vi "MS Operation IOP Ctrl.vi"(6 "PID Cluster":T3={"L1 to L4 PID Cluster"={"L1 PID Gains"={"Kp"=0.005, "Kd"=0.5, "Ki"=0.0005}, "L2 PID Gains"={"Kp"=0.01, "Kd"=1.0, "Ki"=0.005}, "L3 PID Gains"={"Kp"=0.05, "Kd"=1.0, "Ki"=0.0005}, "L4 PID Gains"={"Kp"=0.1, "Kd"=0.1, "Ki"=0.0005}}, "Stage PID Cluster"={"Stage Z PID"={"Kp"=0.0005, "Kd"=0.001, "Ki"=0.0}, "Stage Y PID"={"Kp"=0.0003, "Kd"=0.01, "Ki"=0.0}, "Stage X PID"={"Kp"=0.0003, "Kd"=0.01, "Ki"=0.0}}, "OCT Z PID Gains"={"Kp"=0.0003, "Kd"=0.0001, "Ki"=0.01}}, 8 "error in":errorcluster, 9 "Offset Home 2 RCM":dbl[](array[numeric])=[0.0, 0.0, 0.0, 0.0], 10 "Prev Posit Cluster":T2={"Prev L1 to L4 Posit"=[-0.5319, -0.035669172703475985, -2.0566170657346783, 0.9099264705882353], "Prev Stage Posit"=[6.002553885707208, 5.996566124542428, 5.995469940427586], "Prev OCT Z Posit"=-0.0}, 11 "FPGA VI Reference In":refnum<k20>) -> (0 "error out":errorcluster, 2 "Last Posit Cluster":T1={"Last L1 to L4 Posit"=[0.0, 0.0, 0.0, 0.0], "Last Stage Posit"=[6.0, 6.0, 6.0], "Last OCT Z Posit"=0.0}, 3 "FPGA VI Reference Out":refnum<k20>)   [LabVIEW 2016]
uses:
  <vilib>/Platform/TimedLoop/XDataNode/timing_clust.ctl
  <vilib>/Platform/TimedLoop/XDataNode/nitl_modes.ctl
  <vilib>/Platform/TimedLoop/XDataNode/wakeup.ctl
  Global Variables.vi
  <vilib>/platform/TimedLoop/XDataNode/XDataNode.xnode
  <vilib>/Platform/TimedLoop/XDataNode/XDNodeRunTimeDep.lvlib
  Library/KevinLibraryAll/labview/KevLib01.lvlib
panel:
  out "L1 to L4 Remote cmd":sgl[](array[numeric])
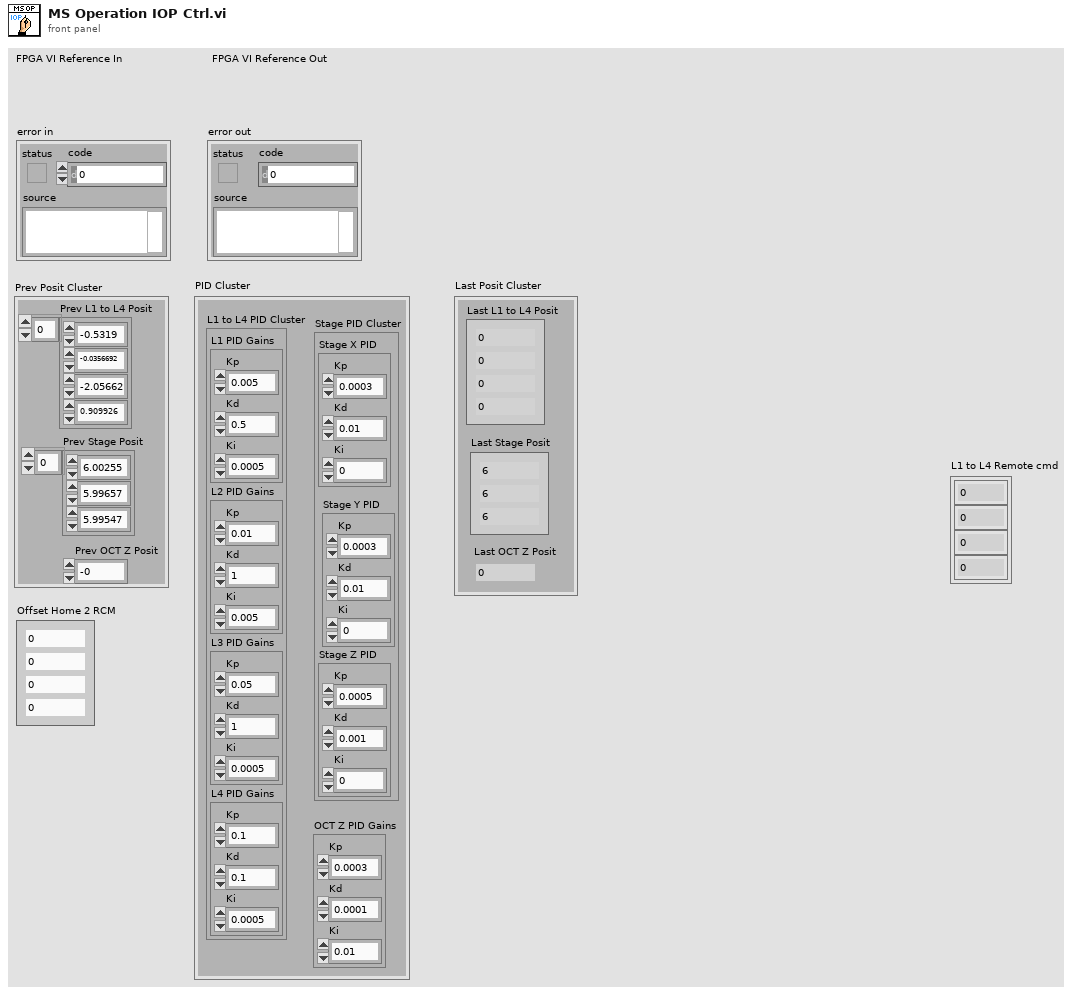
[diagram p1: front panel]
types:
  T1 = cluster{"Last L1 to L4 Posit":dbl[], "Last Stage Posit":dbl[], "Last OCT Z Posit":dbl}
  T2 = cluster{"Prev L1 to L4 Posit":dbl[], "Prev Stage Posit":dbl[], "Prev OCT Z Posit":dbl}
  T3 = cluster{"L1 to L4 PID Cluster":cluster{"L1 PID Gains":cluster{"Kp":dbl, "Kd":dbl, "Ki":dbl}, "L2 PID Gains":cluster{"Kp":dbl, "Kd":dbl, "Ki":dbl}, "L3 PID Gains":cluster{"Kp":dbl, "Kd":dbl, "Ki":dbl}, "L4 PID Gains":cluster{"Kp":dbl, "Kd":dbl, "Ki":dbl}}, "Stage PID Cluster":cluster{"Stage Z PID":cluster{"Kp":dbl, "Kd":dbl, "Ki":dbl}, "Stage Y PID":cluster{"Kp":dbl, "Kd":dbl, "Ki":dbl}, "Stage X PID":cluster{"Kp":dbl, "Kd":dbl, "Ki":dbl}}, "OCT Z PID Gains":cluster{"Kp":dbl, "Kd":dbl, "Ki":dbl}}
  T4 = typedef "XDNodeRunTimeDep.lvlib/timing_clust.ctl" = cluster{"Expected End [f-1]":u64, "Actual End [f-1]":u64, "Finished Late? [f-1]":bool, "Expected End [i-1]":u64, "Actual End [i-1]":u64, "Finished Late? [i-1]":bool, "Expected Start [i]":u64, "Actual Start [i]":u64, "Expected Start [f]":u64, "Actual Start [f]":u64, "Source Name":string, "Structure Name":string, "Period":i64, "Deadline":i64, "Offset":i64, "Start":i64, "Priority":i32, "Timeout":i32, "Mode":T5, "Wakeup Reason":T6, "Error":errorcluster, "Source Type":string, "Secondary Source Type":string, "Global End Time":u64, "Global Start Time":u64, "Frame Duration":u64, "Iteration Duration":u64, "Assigned CPU":i32, "I/O Scan Engine Mode":u32}
  T5 = typedef "XDNodeRunTimeDep.lvlib/nitl_modes.ctl" = enum32{"No Change", "Process missed periods, maintain original phase", "Discard missed periods, maintain original phase", "Process missed periods, ignore original phase", "Discard missed periods, ignore original phase"}
  T6 = typedef "XDNodeRunTimeDep.lvlib/wakeup.ctl" = enum32{"Normal", "Aborted", "Asynchronous wakeup", "Timing source error", "Timed loop error", "Timeout"}
  T7 = cluster{"L1 PID Gains":cluster{"Kp":dbl, "Kd":dbl, "Ki":dbl}, "L2 PID Gains":cluster{"Kp":dbl, "Kd":dbl, "Ki":dbl}, "L3 PID Gains":cluster{"Kp":dbl, "Kd":dbl, "Ki":dbl}, "L4 PID Gains":cluster{"Kp":dbl, "Kd":dbl, "Ki":dbl}}
  T8 = cluster{"Stage Z PID":cluster{"Kp":dbl, "Kd":dbl, "Ki":dbl}, "Stage Y PID":cluster{"Kp":dbl, "Kd":dbl, "Ki":dbl}, "Stage X PID":cluster{"Kp":dbl, "Kd":dbl, "Ki":dbl}}
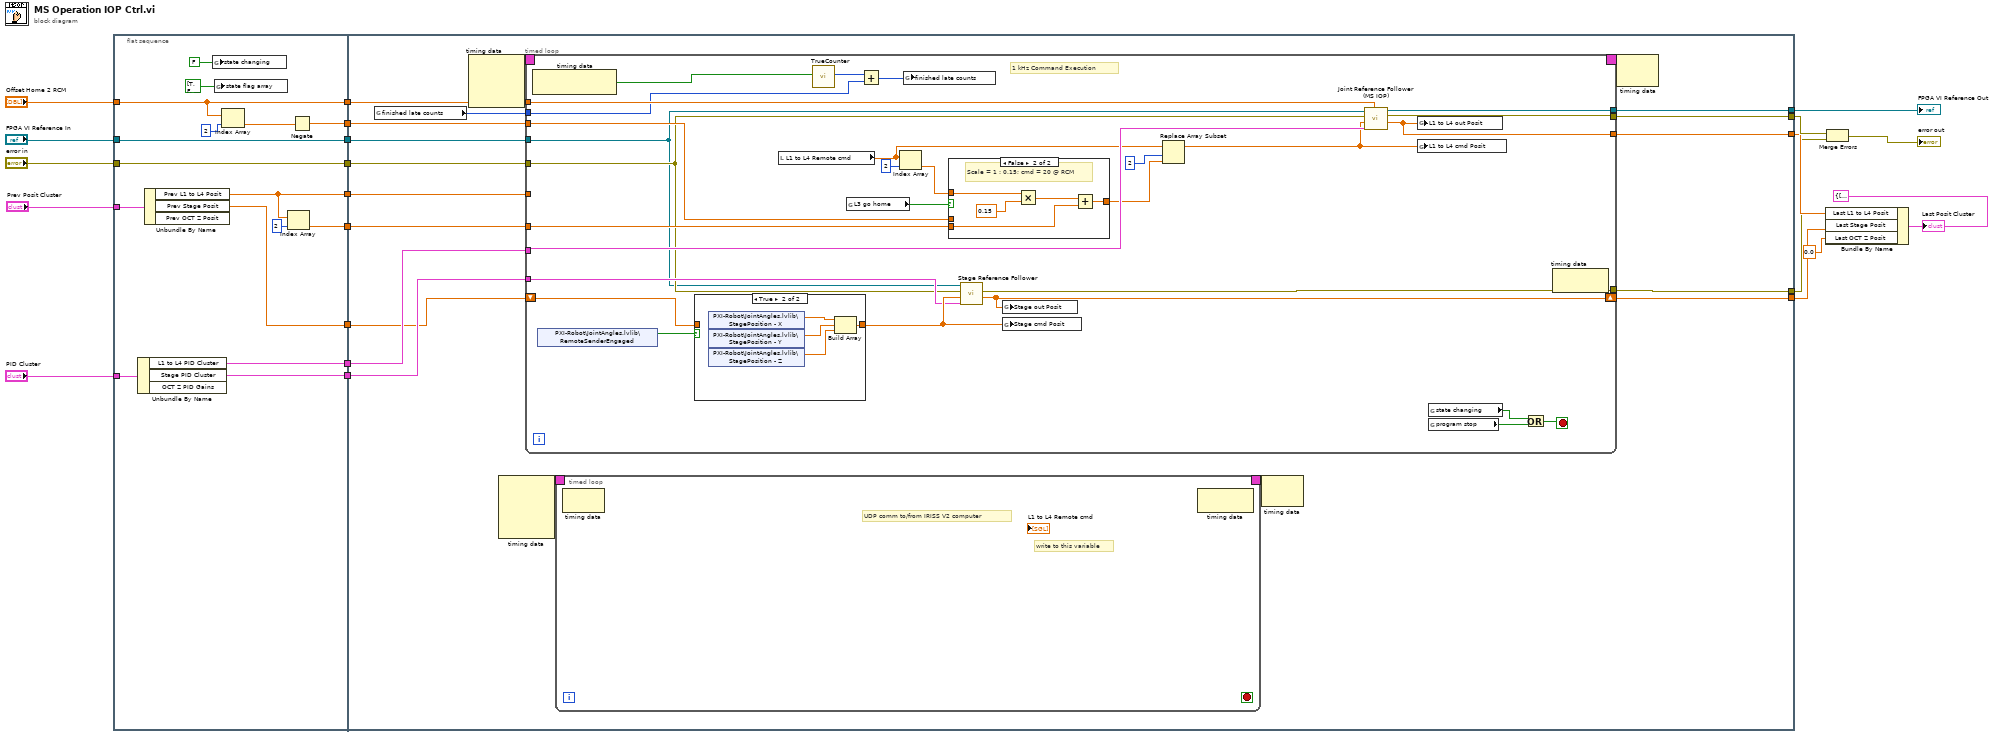
[diagram p0: block diagram]
diagram:
  n1 = flat-sequence {
    tunnel: [w37] -> w23
    tunnel: "FPGA VI Reference In" -> [w37]
    tunnel: [w36] -> w21
    tunnel: "error in" -> [w36]
    tunnel: [w29] -> w19
    tunnel: "Offset Home 2 RCM" -> [w29]
    tunnel: "Prev Posit Cluster" -> [w25]
    tunnel: [w34] -> w16
    tunnel: "PID Cluster" -> [w33]
    tunnel: [w32] -> w14
    tunnel: [w31] -> w13
    tunnel: [w27] -> w12
    tunnel: [w26] -> w3
    tunnel: [w24] -> w2
    tunnel: w23 -> [w43]
    tunnel: w21 -> [w42]
    tunnel: w19 -> [w56]
    tunnel: w16 -> [w55]
    tunnel: w14 -> [w54]
    tunnel: w13 -> [w53]
    tunnel: w12 -> [w52]
    tunnel: [w51] -> w8
    tunnel: [w50] -> w9
    tunnel: [w44] -> w6
    tunnel: [w45] -> w5
    tunnel: [w49] -> w4
    tunnel: w3 -> [w48]
    tunnel: w2 -> [w46]
    frame #0 {
      n2 = Unbundle By Name(w33) -> ("L1 to L4 PID Cluster"=w32:T7, "Stage PID Cluster"=w26:T8)  [unwired: 1 out]
      n3 = Unbundle By Name(w25) -> ("Prev L1 to L4 Posit"=w34:dbl[], "Prev Stage Posit"=w24:dbl[])  [unwired: 1 out]
      n4 = global write "Global Variables.vi" "state changing"(FALSE ("state changing")) -> ()
      n5 = global write "Global Variables.vi" "state flag array"(bool[] [TRUE, FALSE, FALSE, FALSE, FALSE, FALSE, FALSE, FALSE, FALSE] ("state flag array")) -> ()
      n6 = Index Array(array=w29, index=2) -> (element=w28:dbl)
      n7 = Index Array(array=w34, index=2) -> (element=w31:dbl)
      n8 = Negate(x=w28) -> (-x=w27:dbl)
    }
    frame #1 {
      n9 = global read "Global Variables.vi" "finished late counts"() -> (w47:u16)
      n10 = node-c288() -> (w58:T4)  [unwired: 3 in]
      n11 = node-c288() -> (w41:T4)  [unwired: 4 in]
      n12 = timed-loop {
        timing: w58 -> [_]
        timing-out: [_] -> w57
        tunnel: w43 -> [w69]
        tunnel: w42 -> [w70]
        tunnel: w56 -> [w86]
        tunnel: w55 -> [_]
        tunnel: w54 -> [w84]
        tunnel: w53 -> [w83]
        tunnel: w52 -> [w80]
        tunnel: [w79] -> w51
        tunnel: [w78] -> w50
        tunnel: [w77] -> w49
        tunnel: w48 -> [w75]
        tunnel: w47 -> [w71]
        shift-right: [w67] -> w45
        shift-left: w46 -> [w68]
        tunnel: [w64] -> w44
        stop <- w91 stop-if-true
        # "1 kHz Command Execution"
        n13 = node-c288() -> (w74:bool)  [unwired: 1 in]
        n14 = shared-variable "PXI-Robot\\JointAngles.lvlib\\RemoteSenderEngaged"() -> (w66:bool)  [unwired: 1 in, 1 out]
        n15 = case shown="True" w66 {
          tunnel: [w92 w96] -> w85
          tunnel: w68 -> [w92 _]
          frame False {
          }
          frame True {
            n16 = shared-variable "PXI-Robot\\JointAngles.lvlib\\StagePosition - X"() -> (w93:dbl)  [unwired: 1 in, 1 out]
            n17 = shared-variable "PXI-Robot\\JointAngles.lvlib\\StagePosition - Y"() -> (w94:dbl)  [unwired: 1 in, 1 out]
            n18 = shared-variable "PXI-Robot\\JointAngles.lvlib\\StagePosition - Z"() -> (w95:dbl)  [unwired: 1 in, 1 out]
            n19 = Build Array(w93, w94, w95) -> (w96:dbl[])
          }
        }
        n20 = local read "L1 to L4 Remote cmd"() -> (w65:sgl[])
        n21 = call "TrueCounter.vi"("True?"=w74) -> ("True Count"=w72:u16)  [unwired: 10 in]
        n22 = global read "Global Variables.vi" "L3 go home"() -> (w89:bool)
        n23 = Add(x=w72, y=w71) -> (x+y=w73:u16)
        n24 = Index Array(array=w65, index=2) -> (element=w87:sgl)
        n25 = global write "Global Variables.vi" "finished late counts"(w73) -> ()
        n26 = case shown="False" w89 {
          tunnel: [w97 w102] -> w81
          tunnel: w87 -> [_ w99]
          tunnel: w83 -> [_ w98]
          tunnel: w80 -> [w97 _]
          frame True {
            # "Go Home"
          }
          frame False {
            # "Scale = 1 : 0.15; cmd = 20 @ RCM"
            n27 = Multiply(x=w99, y=0.15) -> (x*y=w101:dbl)
            n28 = Add(x=w101, y=w98) -> (x+y=w102:dbl)
          }
        }
        n29 = call "Stage Reference Follower.vi"("Stage PID Cluster"=w75, "Stage cmd Posit [mm]"=w85, "error in"=w70, "FPGA VI Reference In"=w69) -> ("Stage out Posit [mm]"=w67:dbl[], "error out"=w77:errorcluster)  [unwired: 5 in, 1 out]
        n30 = global write "Global Variables.vi" "Stage out Posit"(w67) -> ()
        n31 = global write "Global Variables.vi" "Stage cmd Posit"(w85) -> ()
        n32 = Replace Array Subset(array=w65, new element=w81, index=2) -> (w63:sgl[])
        n33 = call "Joint Reference Follower (MS IOP).vi"("Offset Home2RCM [deg/mm]"=w86, "PID Ctrl Cluster"=w84, "Ref Array [deg/mm]"=w63, "error in"=w70, "FPGA VI Reference In"=w69) -> ("Output Posit Array [deg/mm]"=w64:dbl[], "error out"=w79:errorcluster, "FPGA VI Reference Out"=w78:refnum<k20>)  [unwired: 4 in]
        n34 = global write "Global Variables.vi" "L1 to L4 out Posit"(w64) -> ()
        n35 = global write "Global Variables.vi" "L1 to L4 cmd Posit"(w63) -> ()
        n36 = global read "Global Variables.vi" "state changing"() -> (w90:bool)
        n37 = global read "Global Variables.vi" "program stop"() -> (w76:bool)
        n38 = Or(x=w90, y=w76) -> (x .or. y?=w91:bool)
        n39 = node-c288() -> ()  [unwired: 1 in, 1 out]
      }
      n40 = timed-loop {
        timing: w41 -> [_]
        timing-out: [_] -> w40
        stop <- _ stop-if-true
        # "write to this variable"
        # "UDP comm to/from IRISS V2 computer"
        n41 = node-c288() -> ()  [unwired: 1 in, 1 out]
        n42 = node-c288() -> ()  [unwired: 1 in, 1 out]
      }
      n43 = node-c288(w40) -> ()  [unwired: 1 out]
      n44 = node-c288(w57) -> ()  [unwired: 1 out]
    }
  }
  n45 = Bundle By Name(cluster=T1 {"Last L1 to L4 Posit"=[-0.5607, -0.038216970753724266, -2.0806193533568895, 1.1787683823529411], "Last Stage Posit"=[6.002553885707208, 5.996566124542428, 5.995469940427586], "Last OCT Z Posit"=-0.0} ("Last Posit Cluster 2"), "Last L1 to L4 Posit"=w6, "Last Stage Posit"=w5, "Last OCT Z Posit"=0.0) -> (→"Last Posit Cluster":T1)
  n46 = Merge Errors(w8, w4) -> (→"error out":errorcluster)
  "FPGA VI Reference Out" <- w9
